vi "Get_If_Last_Document.vi"(8 "error in (no error)":errorcluster caption="entrée d'erreur (pas d'erreur)", 11 "Firebase Benches en entrée":refnum<class "Firebase Packaging.lvclass">) -> (0 "error out":errorcluster caption="sortie d'erreur", 2 "Last document ?":bool, 3 "Firebase Benches en sortie":refnum<class "Firebase Packaging.lvclass">)   [LabVIEW 2020, in "Library Instrument & Equipement.lvlib" / "Library FireBase.lvlib" / "Firebase Packaging.lvclass"]
uses:
  Firebase Packaging.lvclass
  Firebase Packaging.lvclass/Firebase Packaging.ctl
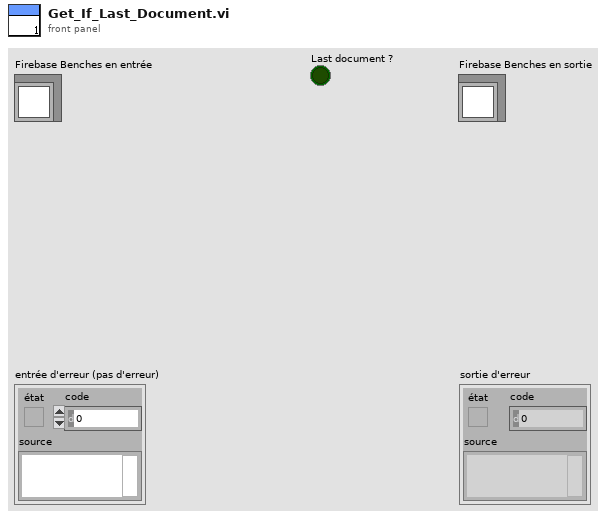
[diagram p1: front panel]
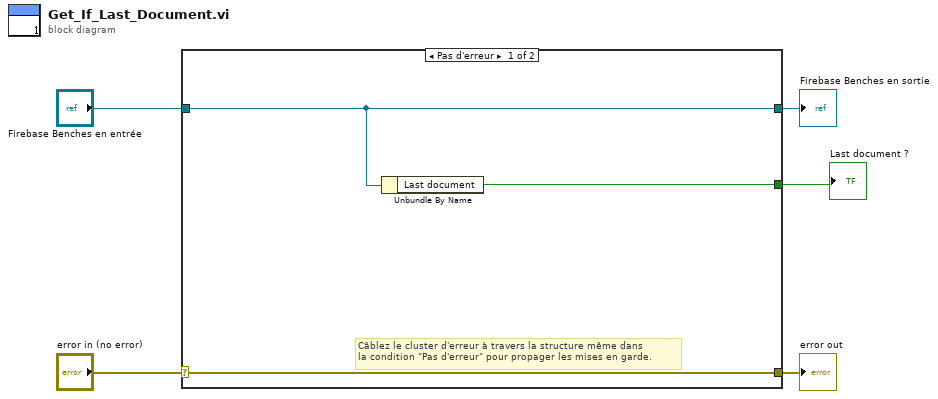
[diagram p0: block diagram]
diagram:
  n1 = case shown="Pas d'erreur" "error in (no error)" {
    selector: "error in (no error)" -> [w8 w10]
    tunnel: [w8 w10] -> w4
    tunnel: [w7 w9] -> w2
    tunnel: "Firebase Benches en entrée" -> [w7 w9]
    tunnel: [w6 _] -> w1
    frame No Error {
      # "Câblez le cluster d'erreur à travers la structure même dans\nla condition \"Pas d'erreur\" pour propager les mises en garde."
      n2 = Unbundle By Name(w7) -> ("Last document"=w6:bool)
    }
    frame Error {
    }
  }
  "error out" <- w4
  "Firebase Benches en sortie" <- w2
  "Last document ?" <- w1
